vi "Write Temperature Set Point (C).vi"(8 "error in (no error)":errorcluster, 10 "Temperature Set Point (C)":dbl, 11 "Thermal Chamber in":refnum<class "Thermal Chamber.lvclass">) -> (0 "error out":errorcluster, 3 "Thermal Chamber out":refnum<class "Thermal Chamber.lvclass">)   [LabVIEW 2016, in "Hardware.lvlib" / "Thermal Chamber.lvclass"]
uses:
  Thermal Chamber.lvclass
  Thermal Chamber.lvclass/Thermal Chamber.ctl
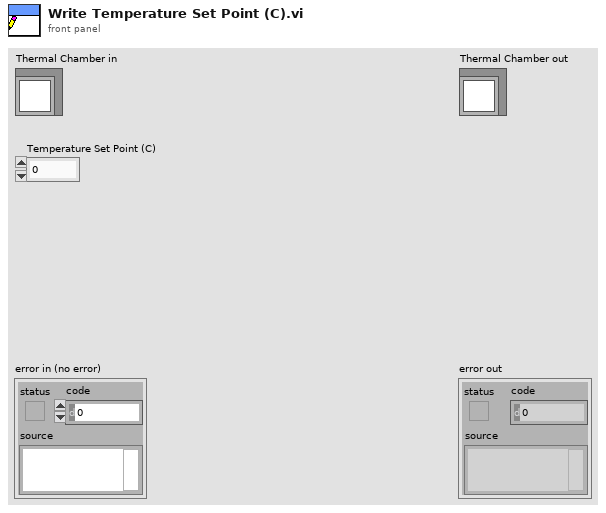
[diagram p1: front panel]
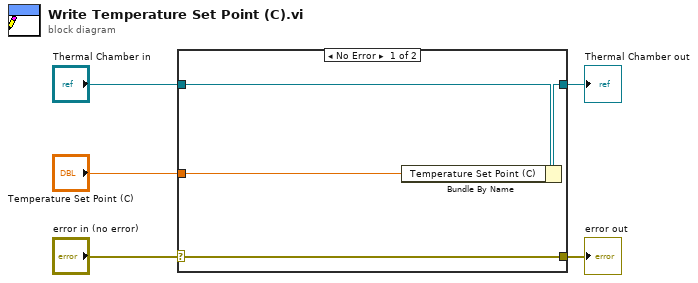
[diagram p0: block diagram]
diagram:
  n1 = case shown="No Error" "error in (no error)" {
    selector: "error in (no error)" -> [w9 w10]
    tunnel: [w9 w10] -> w4
    tunnel: [w7 w11] -> w2
    tunnel: "Thermal Chamber in" -> [w8 w11]
    tunnel: "Temperature Set Point (C)" -> [w6 _]
    frame No Error {
      n2 = Bundle By Name(cluster=w8, "Temperature Set Point (C)"=w6) -> (w7:refnum<class "Thermal Chamber.lvclass">)
    }
    frame Error {
    }
  }
  "error out" <- w4
  "Thermal Chamber out" <- w2
